vi "addAntiConvolutionalLayer.vi"(0 "features":u32, 2 "outBoxes":u32, 4 "func":u32, 5 "stride":u32, 6 "NOUTXY":u32, 7 "kernelXY":u32, 8 "ptr":i64, 9 "error in (no error)":errorcluster) -> (1 "ptr out":i64, 3 "error out":errorcluster)   [LabVIEW 2016, in "CNet.lvlib"]
uses:
  CNet.lvlib
  Users/jg754/Documents/Visual Studio 2015/Projects/CLearn/x64/Release/CLearn.dll
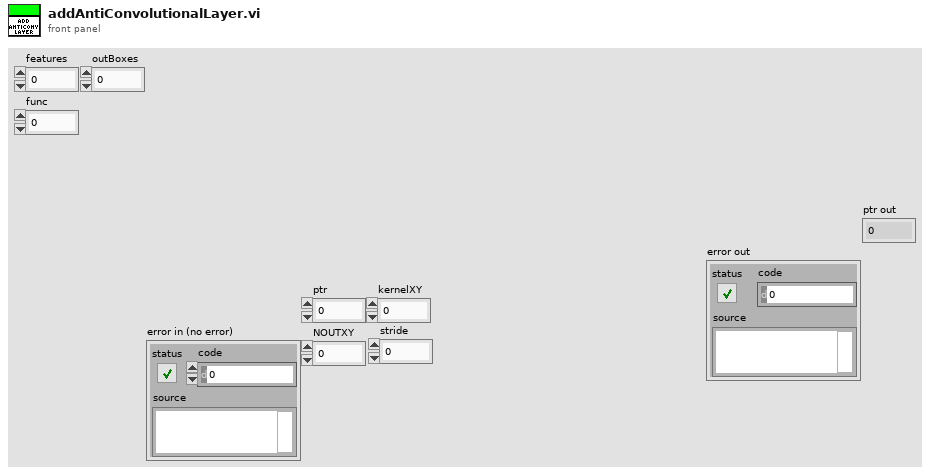
[diagram p1: front panel]
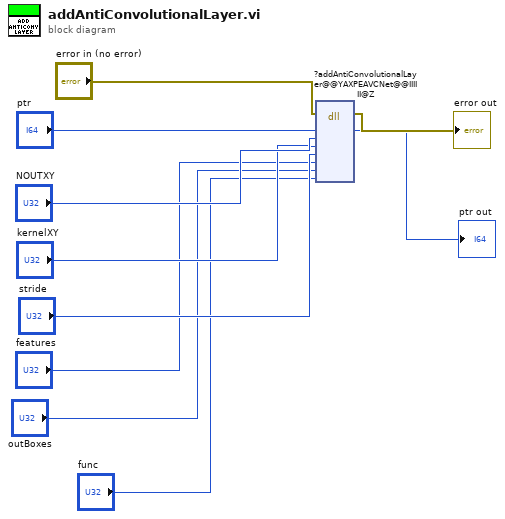
[diagram p0: block diagram]
diagram:
  n1 = dll-call lib="C:/Users/jg754/Documents/Visual Studio 2015/Projects/CLearn/x64/Release/CLearn.dll" fn="?addAntiConvolutionalLayer@@YAXPEAVCNet@@IIIIII@Z"(error in="error in (no error)", "ptr"="ptr", "NOUTXY"="NOUTXY", "kernelXY"="kernelXY", "stride"="stride", "features"="features", "outBoxes"="outBoxes", "func"="func") -> (error out=→"error out":errorcluster, "ptr"=→"ptr out":i64)  [unwired: 9 in, 1 out]
